vi "Einheit changes.vi"(10 "Einheit":T1, 11 "Konzentration in":dbl) -> (3 "Konzentration out":dbl)   [LabVIEW 2020, in "EPA 1065.lvlib" / "HovaCAL Interference verificaton.lvlib"]
uses:
  HovaCAL Interference verificaton.lvlib
  Linearisierung V2/SpanEinstellungen/Einheit.ctl
  Linearisierung V2/SpanEinstellungen/SpanEinstellungen.lvlib
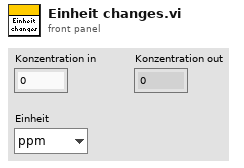
[diagram p1: front panel]
types:
  T1 = typedef "Linearisierung v2.lvlib/SpanEinstellungen.lvlib/Einheit.ctl" = enum16{"ppm", "%"}
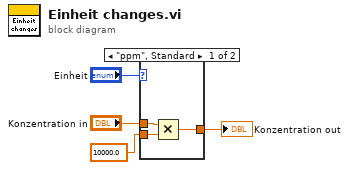
[diagram p0: block diagram]
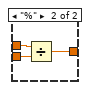
[diagram p2: hidden frame]
diagram:
  n1 = case shown="\"ppm\", Standard" "Einheit" {
    tunnel: "Konzentration in" -> [w7 w10]
    tunnel: [w6 w8] -> w4
    tunnel: 10000.0 ("y") -> [w5 w9]
    frame "ppm", Default {
      n2 = Multiply(x=w7, y=w5) -> (x*y=w6:dbl)
    }
    frame "%" {
      n3 = Divide(x=w10, y=w9) -> (x/y=w8:dbl)
    }
  }
  "Konzentration out" <- w4
